vi "Set RTD Props.vi"(8 "error in (no error)":errorcluster, 10 "temp param":T1={"A"=0.00139999995008111, "B"=0.00023700000019744039, "C"=9.899999753315569e-08, "R0"=1000.0}, 11 "Item Ref in":T2 format="%.0x") -> (0 "error out":errorcluster, 3 "Item Ref out":T2 format="%.0x")   [LabVIEW 2011, in "NI 272x Resistive Simulation Custom Device Configuration.lvlib"]
uses:
  NI 272x Resistive Simulation Custom Device Configuration.lvlib
  <vilib>/NI Veristand/Custom Device API/Custom Device Item Ref.ctl
  <instrlib>/ni272xReferenceVIs/ni272xReferenceVIs.llb/ni272x Callendar-Van Dusen RTD Parameters.ctl
  Globals/Names.vi
  <vilib>/NI Veristand/Custom Device API/Set Item Property (Double).vi
  <vilib>/NI Veristand/Custom Device API/Custom Device API.lvlib
  NI 272x Resistive Simulation Custom Device Shared.lvlib
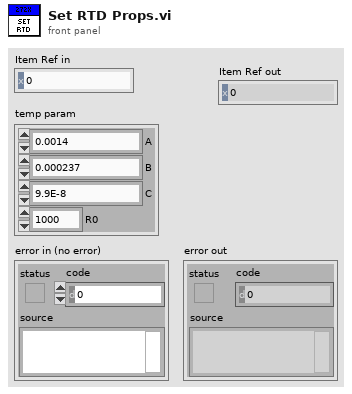
[diagram p1: front panel]
types:
  T1 = typedef "ni272x Callendar-Van Dusen RTD Parameters.ctl" = cluster{"A":dbl, "B":dbl, "C":dbl, "R0":dbl}
  T2 = typedef "Custom Device API.lvlib/Custom Device Item Ref.ctl" = u64
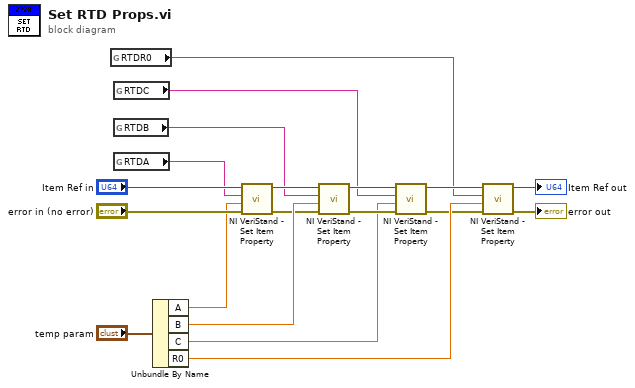
[diagram p0: block diagram]
diagram:
  n1 = global read "Names.vi" "RTDR0"() -> (w7:string)
  n2 = global read "Names.vi" "RTDC"() -> (w8:string)
  n3 = global read "Names.vi" "RTDB"() -> (w9:string)
  n4 = global read "Names.vi" "RTDA"() -> (w17:string)
  n5 = Unbundle By Name("temp param") -> ("A"=w15:dbl, "B"=w6:dbl, "C"=w3:dbl, "R0"=w2:dbl)
  n6 = call-poly <vilib>:"NI VeriStand - Set Item Property.vi"("error in (no error)"="error in (no error)", "Value"=w15, "Property Name"=w17, "Item Ref in"="Item Ref in") -> ("error out"=w5:errorcluster, "Item Ref out"=w14:T2)  [unwired: 5 in, 1 out]
  n7 = call-poly <vilib>:"NI VeriStand - Set Item Property.vi"("error in (no error)"=w5, "Value"=w6, "Property Name"=w9, "Item Ref in"=w14) -> ("error out"=w4:errorcluster, "Item Ref out"=w13:T2)  [unwired: 5 in, 1 out]
  n8 = call-poly <vilib>:"NI VeriStand - Set Item Property.vi"("error in (no error)"=w4, "Value"=w3, "Property Name"=w8, "Item Ref in"=w13) -> ("error out"=w1:errorcluster, "Item Ref out"=w12:T2)  [unwired: 5 in, 1 out]
  n9 = call-poly <vilib>:"NI VeriStand - Set Item Property.vi"("error in (no error)"=w1, "Value"=w2, "Property Name"=w7, "Item Ref in"=w12) -> ("error out"=→"error out":errorcluster, "Item Ref out"=→"Item Ref out":T2)  [unwired: 5 in, 1 out]
